vi "VISA Test.vi"(8 "error in":errorcluster, 11 "VISA resource name":refnum<visa-resource-name>) -> (0 "error out":errorcluster, 3 "VISA resource name out":refnum<visa-resource-name>)   [LabVIEW 2020, in "ChromTech MX-Class Drivers.lvlib"]
doc: "Simple VI designed to test VISA communication to the instrument. This application opens a session to the instrument, performs a write of the fetch ID command \"ID\\r\", and queries the device for its response."
uses:
  <instrlib>/RxnRover/ChromtechNextGenDriver/ChromTech MX-Class Drivers.lvlib
panel:
  in  "Fast Comms":bool
  out "Instrument Response":string
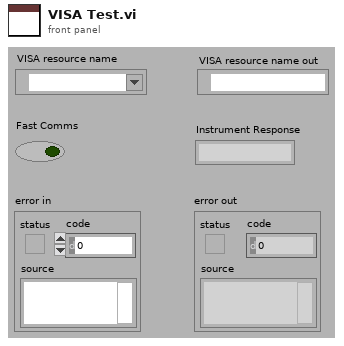
[diagram p1: front panel]
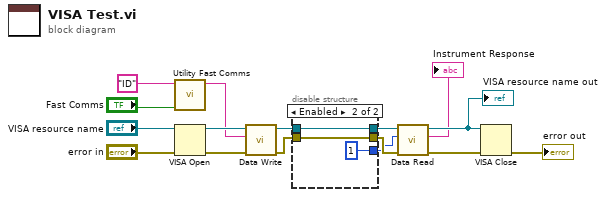
[diagram p0: block diagram]
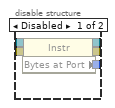
[diagram p2: hidden frame]
diagram:
  n1 = call <instrlib>:"Utility Fast Comms.vi"("Fast Comms"="Fast Comms", "Command"="ID") -> ("Fast Command"=w6:string)  [unwired: 9 in]
  n2 = VISA Open(error in (no error)="error in", VISA resource name="VISA resource name") -> (VISA resource name=w14:refnum<visa-resource-name>, error out=w13:errorcluster)  [unwired: 3 in]
  n3 = call <instrlib>:"Data Write.vi"("error in (no error)"=w13, "Command"=w6, "VISA Refnum in"=w14) -> ("error out"=w3:errorcluster, "VISA Refnum out"=w5:refnum<visa-resource-name>)  [unwired: 7 in]
  n4 = disable-structure shown="Enabled" {
    disable-tunnel: w5 -> [w21 w24]
    disable-tunnel: [w20 w24] -> w4
    disable-tunnel: w3 -> [w19 w23]
    disable-tunnel: [w18 w23] -> w2
    disable-tunnel: [w17 1] -> w1
    frame Disabled {
      n5 = property class="Instr"(reference=w21, error in=w19) -> (reference out=w20:refnum<visa-resource-name>, error out=w18:errorcluster, "Bytes at Port"=w17:u32)
    }
    frame Enabled {
    }
  }
  n6 = call <instrlib>:"Data Read.vi"("error in (no error)"=w2, "Bytes to read"=w1, "VISA Refnum in"=w4) -> ("error out"=w12:errorcluster, "read buffer"=→"Instrument Response":string, "VISA Refnum out"=w10:refnum<visa-resource-name>)  [unwired: 6 in]
  "VISA resource name out" <- w10
  n7 = VISA Close(VISA resource name=w10, error in (no error)=w12) -> (error out=→"error out":errorcluster)
